vi "HAL camera calculate binning.vi"(11 "Camera Parameters (important)":T1 {"Image Size"."Binning" items=["1 x 1"=1, "2 x 2"=2, "4 x 4"=4]; "Image Size"."Bottom" min=4 max=2048 step=4; "Image Size"."Right" min=4 max=2048 step=4; "Image Size"."Top" min=1 max=2048 step=4; "Image Size"."Left" min=1 max=2048 step=4; "Exposure Time (sec)" scale=0.001..10.0 scale format="%#_1g"}) -> (2 "V Bin":i32, 3 "H Bin":i32)   [LabVIEW 2011]
uses:
  HAL camera parameters important.ctt
  orca readout settings.ctl
  image size.ctl
panel:
  # "Camera: Hammamatsu Orca"
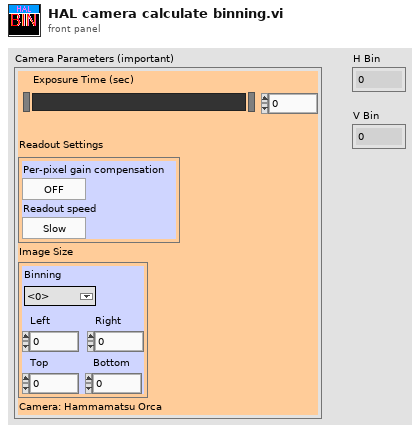
[diagram p1: front panel]
types:
  T1 = typedef "HAL camera parameters important.ctt" = cluster{"Exposure Time (sec)":sgl, "Readout Settings":T2, "Image Size":T3}
  T2 = typedef "orca readout settings.ctl" = cluster{"Per-pixel gain compensation":bool, "Readout speed":bool}
  T3 = typedef "image size.ctl" = cluster{"Left":i32, "Top":i32, "Right":i32, "Bottom":i32, "Binning":u16}
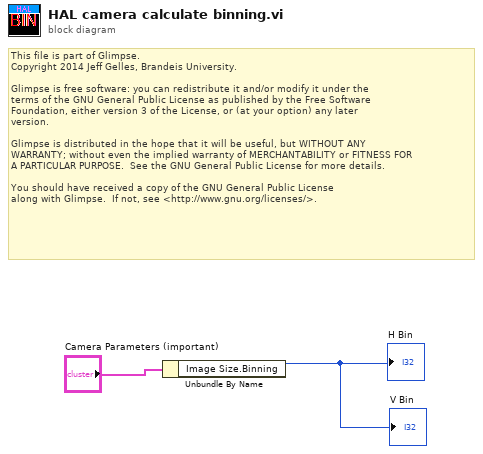
[diagram p0: block diagram]
diagram:
  # "This file is part of Glimpse. \nCopyright 2014 Jeff Gelles, Brandeis University.    \n\nGlimpse is free software: you can redistribute it and/or modify it under the \nterms of the GNU General Public License as published by the Free Software \nFoundation, either version 3 of the License, or (at your option) any later \nversion.\n\nGlimpse is distributed in the hope that it will be useful, but WITHOUT ANY \nWARRANTY; without even the implied warranty of MERCHANTABILITY or FITNESS FOR \nA PARTICULAR PURPOSE.  See the GNU General Public License for more details.\n\nYou should have received a copy of the GNU General Public License\nalong with Glimpse.  If not, see <http://www.gnu.org/licenses/>."
  n1 = Unbundle By Name("Camera Parameters (important)") -> ("Image Size.Binning"=→"V Bin" →"H Bin":u16)
